vi "Two Character Display.vi"() -> ()   [LabVIEW 2014]
uses:
  <vilib>/myRIO/Instrument Drivers/Onboard IO/DIO/typedefs/DIO Reference.ctl
  <vilib>/myRIO/Common/Instrument Driver Framework/Utilities/typedefs/myRIO Generic Hardware Reference.ctl
  <vilib>/myRIO/Common/Instrument Driver Framework/Utilities/typedefs/Hardware Version Enum.ctl
  <vilib>/myRIO/Common/Instrument Driver Framework/Utilities/typedefs/myRIO v1.0 Reference.ctl
  <vilib>/myRIO/Common/Instrument Driver Framework/Utilities/typedefs/Generic FPGA Reference.ctl
  <vilib>/myRIO/Common/Instrument Driver Framework/myRIO v1.0/DIO/typedefs/DIO Channels List.ctl
  <vilib>/myRIO/Common/Instrument Driver Framework/myRIO v1.0/DIO/typedefs/DIO Channels Enum.ctl
  <vilib>/userdefined/High Color/nirio_resource_hc.ctl
  <vilib>/myRIO/Common/Instrument Driver Framework/Utilities/vis/Is FPGA Ref Available.vi
  <vilib>/myRIO/Common/Instrument Driver Framework/myRIO v1.0/DIO/vis/myRIO v1.1 Open DIO.vi
  <vilib>/myRIO/Instrument Drivers/Onboard IO/DIO/vis/Write.vi
  <vilib>/myRIO/Common/Instrument Driver Framework/Utilities/vis/Validate Channels.vi
  <vilib>/myRIO/Common/Instrument Driver Framework/myRIO v1.0/DIO/vis/myRIO v1.0 Reserve DIO.vi
  <vilib>/myRIO/Common/Instrument Driver Framework/myRIO v1.0/Resource Manager/vis/myRIO v1.0 Reserve Channel List.vi
  <vilib>/myRIO/Common/Instrument Driver Framework/myRIO v1.0/DIO/vis/myRIO v1.0 Build MUX Configuration DIO.vi
  <vilib>/myRIO/Common/Instrument Driver Framework/myRIO v1.0/Resource Manager/vis/myRIO v1.0 Reserve Channel.vi
  <vilib>/myRIO/Common/Instrument Driver Framework/myRIO v1.0/Resource Manager/vis/myRIO v1.0 Unreserve Channel.vi
  <vilib>/myRIO/Common/Instrument Driver Framework/myRIO v1.0/Resource Manager/vis/myRIO v1.0 Create Configuration List.vi
  <vilib>/myRIO/Common/Instrument Driver Framework/myRIO v1.0/Resource Manager/vis/myRIO v1.0 Build Mutex Name.vi
  <vilib>/Utility/VariantDataType/GetNumericInfo.vi
  <vilib>/Utility/error.llb/Error Cluster From Error Code.vi
  <vilib>/myRIO/Common/Instrument Driver Framework/myRIO v1.0/myRIO v1.1 Open.vi
  <vilib>/myRIO/Common/Instrument Driver Framework/Utilities/vis/IO Manager.vi
  <vilib>/myRIO/Common/Instrument Driver Framework/Utilities/vis/Configuration Manager.vi
  <vilib>/myRIO/Common/Instrument Driver Framework/myRIO v1.0/Resource Manager/vis/myRIO v1.0 Configure IO.vi
  <vilib>/myRIO/Common/Instrument Driver Framework/myRIO v1.0/myRIO v1.0 Close.vi
  <vilib>/myRIO/Common/Instrument Driver Framework/myRIO v1.0/DIO/vis/myRIO v1.0 Write DIO.vi
  <vilib>/myRIO/Express VI/Onboard IO/DO/DO Express VI.xnode
  <vilib>/myRIO/Instrument Drivers/Onboard IO/DIO/vis/myRIO DIO Open.xnode
  <vilib>/myRIO/Instrument Drivers/Onboard IO/DIO/DIO.lvlib
panel:
  out "Second Tens":bool[](array[boolean]) caption="Seconds"
  out "Second Ones":bool[](array[boolean])
  out "Minute Ones":bool[](array[boolean])
  out "Minute Tens":bool[](array[boolean]) caption="Minutes"
  in  "Stop Button":bool
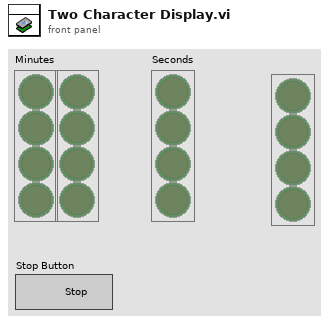
[diagram p1: front panel]
types:
  T1 = typedef "DIO.lvlib/DIO Reference.ctl" = cluster{"myRIO Reference":T2, "DIO Channels List":T6}
  T2 = typedef "myRIO Generic Hardware Reference.ctl" = cluster{"myRIO Model":T3, "myRIO Hardware Reference":T4}
  T3 = typedef "Hardware Version Enum.ctl" = enum16{"Unknown", "myRIO-1900", "myRIO-1950"}
  T4 = typedef "myRIO v1.0 Reference.ctl" = cluster{"Generic FPGA Reference":T5, "Allow multiple opens":bool}
  T5 = typedef "Generic FPGA Reference.ctl" = refnum<k20>
  T6 = typedef "DIO Channels List.ctl" = T7[]
  T7 = typedef "DIO Channels Enum.ctl" = enum16{"Not Connected", "C/DIO0", "C/DIO1", "C/DIO2", "C/DIO3", "C/DIO4", "C/DIO5", "C/DIO6", "C/DIO7", "A/DIO0", "A/DIO1", "A/DIO2", "A/DIO3", "A/DIO4", "A/DIO5", "A/DIO6", "A/DIO7", "A/DIO8", "A/DIO9", "A/DIO10", "A/DIO11", "A/DIO12", "A/DIO13", "A/DIO14", "A/DIO15", "B/DIO0", "B/DIO1", "B/DIO2", "B/DIO3", "B/DIO4", "B/DIO5", "B/DIO6", "B/DIO7", "B/DIO8", "B/DIO9", "B/DIO10", "B/DIO11", "B/DIO12", "B/DIO13", "B/DIO14", "B/DIO15", "LED0", "LED1", "LED2", "LED3", "Button0"}
  T8 = typedef "nirio_resource_hc.ctl" = tag
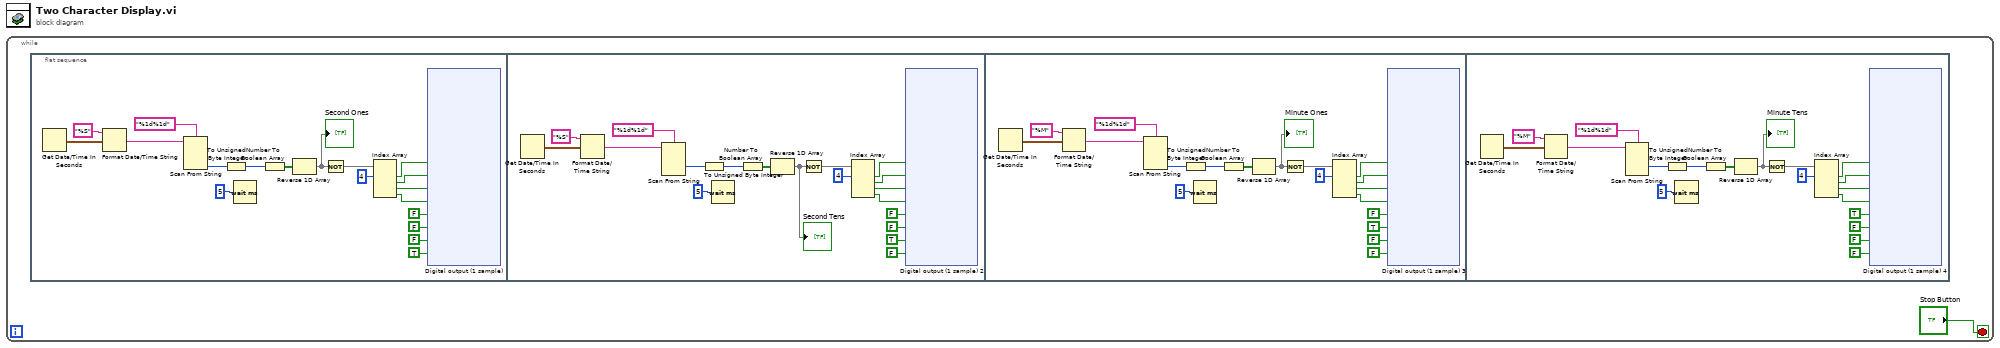
[diagram p0: block diagram]
diagram:
  n1 = while {
    stop <- "Stop Button" stop-if-true
    n2 = flat-sequence {
      frame #0 {
        n3 = Get Date/Time In Seconds() -> (seconds since 1Jan1904=w18:timestamp)
        n4 = Format Date/Time String(time format string (%c)="%S", seconds (now)=w18) -> (date/time string=w17:string)  [unwired: 1 in]
        n5 = Scan From String(format string="%1d%1d", input string=w17) -> (output 2=w15:i32)  [unwired: 5 in, 3 out]
        n6 = To Unsigned Byte Integer(number=w15) -> (unsigned 8bit integer=w16:u8)
        n7 = Wait (ms)(milliseconds to wait=u32 5) -> ()  [unwired: 1 out]
        n8 = Number To Boolean Array(number=w16) -> (Boolean array=w5:bool[])
        n9 = Reverse 1D Array(array=w5) -> (reversed array=w3:bool[])
        "Second Ones" <- w3
        n10 = Not(x=w3) -> (.not. x?=w4:bool[])
        n11 = Index Array(array=w4, index #1=4 ("index")) -> (element #1=w9:bool, element #2=w8:bool, element #3=w7:bool, element #4=w6:bool)  [unwired: 3 in]
        n12 = xnode "Digital output (1 sample)"("B/DIO0 (Pin 11)"=w9, "B/DIO1 (Pin 13)"=w8, "B/DIO2 (Pin 15)"=w7, "B/DIO3 (Pin 17)"=w6, "B/DIO4 (Pin 19)"=FALSE ("B/DIO7 (Pin 25)"), "B/DIO5 (Pin 21)"=FALSE ("B/DIO7 (Pin 25)"), "B/DIO6 (Pin 23)"=FALSE ("B/DIO7 (Pin 25)"), "B/DIO7 (Pin 25)"=TRUE) -> ()  [unwired: 1 in, 1 out]
      }
      frame #1 {
        n13 = Get Date/Time In Seconds() -> (seconds since 1Jan1904=w80:timestamp)
        n14 = Format Date/Time String(time format string (%c)="%S", seconds (now)=w80) -> (date/time string=w81:string)  [unwired: 1 in]
        n15 = Scan From String(format string="%1d%1d", input string=w81) -> (output 1=w78:i32)  [unwired: 5 in, 3 out]
        n16 = To Unsigned Byte Integer(number=w78) -> (unsigned 8bit integer=w77:u8)
        n17 = Wait (ms)(milliseconds to wait=u32 5) -> ()  [unwired: 1 out]
        n18 = Number To Boolean Array(number=w77) -> (Boolean array=w66:bool[])
        n19 = Reverse 1D Array(array=w66) -> (reversed array=w65:bool[])
        "Second Tens" <- w65
        n20 = Not(x=w65) -> (.not. x?=w64:bool[])
        n21 = Index Array(array=w64, index #1=4 ("index")) -> (element #1=w70:bool, element #2=w69:bool, element #3=w68:bool, element #4=w67:bool)  [unwired: 3 in]
        n22 = xnode "Digital output (1 sample) 2"("B/DIO0 (Pin 11)"=w70, "B/DIO1 (Pin 13)"=w69, "B/DIO2 (Pin 15)"=w68, "B/DIO3 (Pin 17)"=w67, "B/DIO4 (Pin 19)"=FALSE ("B/DIO7 (Pin 25)"), "B/DIO5 (Pin 21)"=FALSE ("B/DIO7 (Pin 25)"), "B/DIO6 (Pin 23)"=TRUE ("B/DIO7 (Pin 25)"), "B/DIO7 (Pin 25)"=FALSE) -> ()  [unwired: 1 in, 1 out]
      }
      frame #2 {
        n23 = Get Date/Time In Seconds() -> (seconds since 1Jan1904=w141:timestamp)
        n24 = Format Date/Time String(time format string (%c)="%M", seconds (now)=w141) -> (date/time string=w139:string)  [unwired: 1 in]
        n25 = Scan From String(format string="%1d%1d", input string=w139) -> (output 2=w136:i32)  [unwired: 5 in, 3 out]
        n26 = To Unsigned Byte Integer(number=w136) -> (unsigned 8bit integer=w138:u8)
        n27 = Wait (ms)(milliseconds to wait=u32 5) -> ()  [unwired: 1 out]
        n28 = Number To Boolean Array(number=w138) -> (Boolean array=w137:bool[])
        n29 = Reverse 1D Array(array=w137) -> (reversed array=w124:bool[])
        "Minute Ones" <- w124
        n30 = Not(x=w124) -> (.not. x?=w126:bool[])
        n31 = Index Array(array=w126, index #1=4 ("index")) -> (element #1=w130:bool, element #2=w129:bool, element #3=w128:bool, element #4=w127:bool)  [unwired: 3 in]
        n32 = xnode "Digital output (1 sample) 3"("B/DIO0 (Pin 11)"=w130, "B/DIO1 (Pin 13)"=w129, "B/DIO2 (Pin 15)"=w128, "B/DIO3 (Pin 17)"=w127, "B/DIO4 (Pin 19)"=FALSE ("B/DIO7 (Pin 25)"), "B/DIO5 (Pin 21)"=TRUE ("B/DIO7 (Pin 25)"), "B/DIO6 (Pin 23)"=FALSE ("B/DIO7 (Pin 25)"), "B/DIO7 (Pin 25)"=FALSE) -> ()  [unwired: 1 in, 1 out]
      }
      frame #3 {
        n33 = Get Date/Time In Seconds() -> (seconds since 1Jan1904=w201:timestamp)
        n34 = Format Date/Time String(time format string (%c)="%M", seconds (now)=w201) -> (date/time string=w203:string)  [unwired: 1 in]
        n35 = Scan From String(format string="%1d%1d", input string=w203) -> (output 1=w198:i32)  [unwired: 5 in, 3 out]
        n36 = To Unsigned Byte Integer(number=w198) -> (unsigned 8bit integer=w199:u8)
        n37 = Wait (ms)(milliseconds to wait=u32 5) -> ()  [unwired: 1 out]
        n38 = Number To Boolean Array(number=w199) -> (Boolean array=w197:bool[])
        n39 = Reverse 1D Array(array=w197) -> (reversed array=w185:bool[])
        "Minute Tens" <- w185
        n40 = Not(x=w185) -> (.not. x?=w187:bool[])
        n41 = Index Array(array=w187, index #1=4 ("index")) -> (element #1=w191:bool, element #2=w190:bool, element #3=w189:bool, element #4=w188:bool)  [unwired: 3 in]
        n42 = xnode "Digital output (1 sample) 4"("B/DIO0 (Pin 11)"=w191, "B/DIO1 (Pin 13)"=w190, "B/DIO2 (Pin 15)"=w189, "B/DIO3 (Pin 17)"=w188, "B/DIO4 (Pin 19)"=TRUE ("B/DIO7 (Pin 25)"), "B/DIO5 (Pin 21)"=FALSE ("B/DIO7 (Pin 25)"), "B/DIO6 (Pin 23)"=FALSE ("B/DIO7 (Pin 25)"), "B/DIO7 (Pin 25)"=FALSE) -> ()  [unwired: 1 in, 1 out]
      }
    }
  }
